vi "S7-TCP_Write.vi"(5 "DataType":T1=enum."Dword", 7 "DB #":u16=1, 8 "error in (no error)":errorcluster caption="错误输入（无错误）", 9 "WriteData":sgl[](array[numeric]), 10 "WriteAddress":sgl format="%#.1g", 11 "S7-TCP 输入":refnum<class "S7-TCP.lvclass">) -> (0 "error out":errorcluster caption="错误输出", 2 "Data Valid":bool, 3 "S7-TCP 输出":refnum<class "S7-TCP.lvclass">)   [LabVIEW 2018, in "S7-TCP.lvclass"]
uses:
  S7-TCP.lvclass
  Controls/WriteDataType.ctl
  Controls/RegisterType.ctl
  S7-TCP.lvclass/S7-TCP.ctl
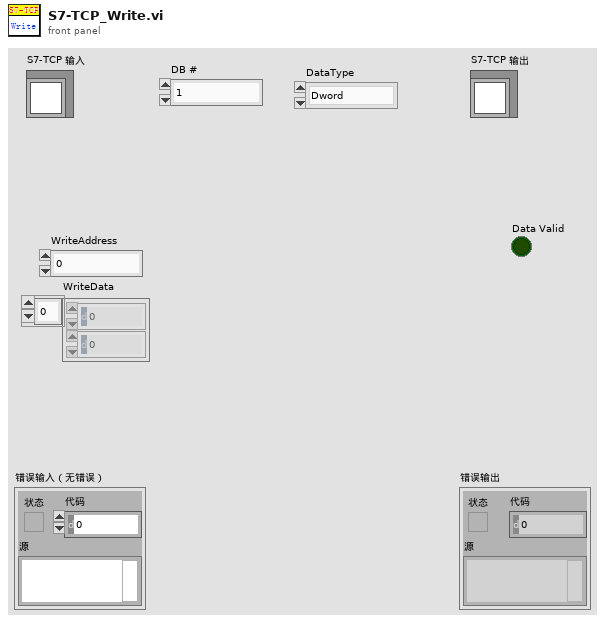
[diagram p1: front panel]
types:
  T1 = typedef "S7-TCP.lvclass/WriteDataType.ctl" = enum16{"Byte", "Word", "Dword", "Real", "Bit"}
  T2 = typedef "S7-TCP.lvclass/RegisterType.ctl" = u8
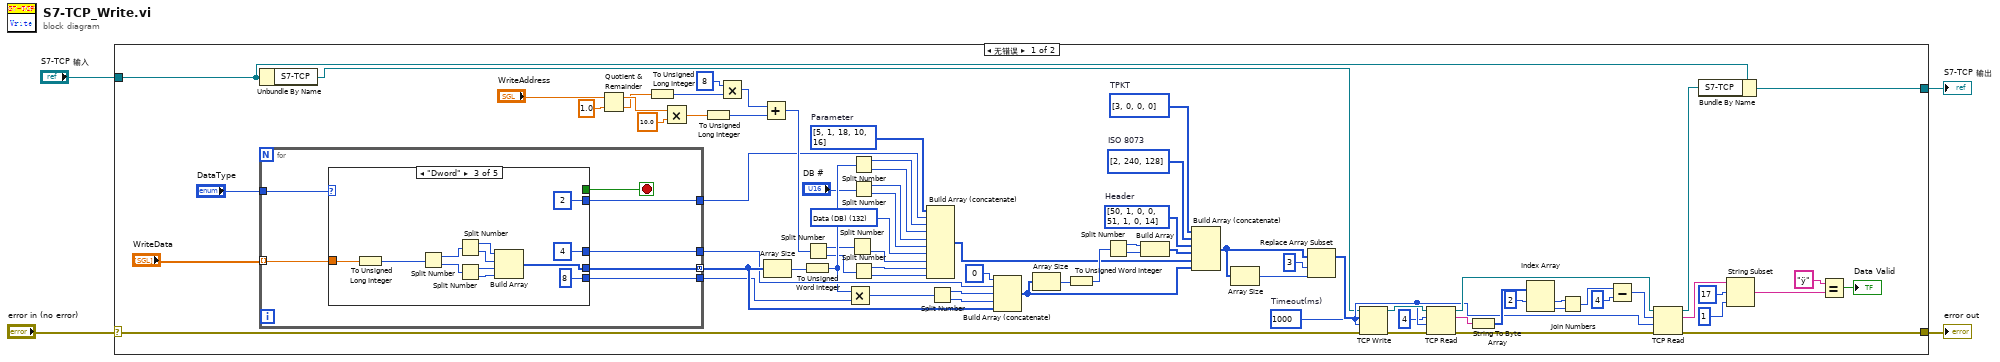
[diagram p0: block diagram]
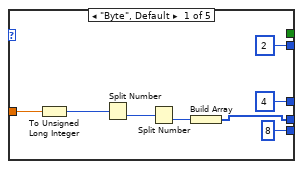
[diagram p2: hidden frame]
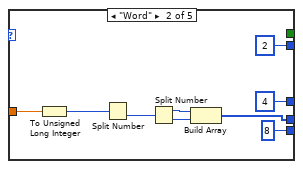
[diagram p3: hidden frame]
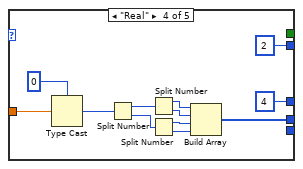
[diagram p4: hidden frame]
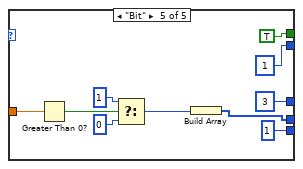
[diagram p5: hidden frame]
diagram:
  n1 = case shown="无错误" "error in (no error)" {
    selector: "error in (no error)" -> [w9 w139]
    tunnel: [w5 w139] -> w3
    tunnel: [w7 w138] -> w1
    tunnel: "S7-TCP 输入" -> [w79 w138]
    frame No Error {
      w12 = T2 132 items=["I/O (P)"=128, "Input (I)"=129, "Output (Q)"=130, "Bit Memory (M)"=131, "Data (DB)"=132, "Instance Data (DI)"=133, "Local Data (L)"=134, "Predecessor Local Data (VL)"=135] ("RegisterType")
      w24 = u32 1000  # Timeout(ms)
      w16 = u8[] [50, 1, 0, 0, 51, 1, 0, 14]  # Header
      w18 = u8[] [3, 0, 0, 0]  # TPKT
      w17 = u8[] [2, 240, 128]  # ISO 8073
      w13 = u8[] [5, 1, 18, 10, 16]  # Parameter
      n2 = Unbundle By Name(w79) -> ("S7-TCP"=w8:refnum<k5>)
      n3 = for {
        tunnel: "DataType" -> [w86]
        tunnel: "WriteData" -> [w85] mode=indexing
        tunnel: [w80] -> w78 mode=concatenating
        tunnel: [w84] -> w49
        tunnel: [w83] -> w63
        tunnel: [w82] -> w64
        stop <- w81 stop-if-true
        n4 = case shown="\"Dword\"" w86 {
          tunnel: w85 -> [w93 w100 w108 w118 w137]
          tunnel: [w94 w103 w109 w119 w132] -> w80
          tunnel: [u8 2 ("Numeric") u8 2 ("Numeric") u8 2 ("Numeric") u8 2 ("Numeric") u8 1 ("Numeric")] -> w84
          tunnel: [u8 4 ("Numeric") u8 4 ("Numeric") u8 4 ("Numeric") u8 4 ("Numeric") u8 3 ("Numeric")] -> w83
          tunnel: [u8 8 ("y") u8 8 ("y") u8 8 ("y") _ u16 1 ("y")] -> w82
          tunnel: [_ _ _ _ TRUE] -> w81
          frame "Byte", Default {
            n5 = To Unsigned Long Integer(number=w93) -> (unsigned 32bit integer=w91:u32)
            n6 = Split Number(x=w91) -> (lo(x)=w92:u16)  [unwired: 1 out]
            n7 = Split Number(x=w92) -> (lo(x)=w90:u8)  [unwired: 1 out]
            n8 = Build Array(w90) -> (w94:u8[])
          }
          frame "Word" {
            n9 = To Unsigned Long Integer(number=w100) -> (unsigned 32bit integer=w99:u32)
            n10 = Split Number(x=w99) -> (lo(x)=w98:u16)  [unwired: 1 out]
            n11 = Split Number(x=w98) -> (hi(x)=w102:u8, lo(x)=w101:u8)
            n12 = Build Array(w102, w101) -> (w103:u8[])
          }
          frame "Dword" {
            n13 = To Unsigned Long Integer(number=w108) -> (unsigned 32bit integer=w107:u32)
            n14 = Split Number(x=w107) -> (hi(x)=w115:u16, lo(x)=w114:u16)
            n15 = Split Number(x=w115) -> (hi(x)=w113:u8, lo(x)=w112:u8)
            n16 = Split Number(x=w114) -> (hi(x)=w111:u8, lo(x)=w110:u8)
            n17 = Build Array(w113, w112, w111, w110) -> (w109:u8[])
          }
          frame "Real" {
            n18 = Type Cast ("强制类型转换")(type=u32 0, x=w118) -> (*(type *) &x=w124:u32)
            n19 = Split Number(x=w124) -> (hi(x)=w126:u16, lo(x)=w125:u16)
            n20 = Split Number(x=w126) -> (hi(x)=w123:u8, lo(x)=w122:u8)
            n21 = Split Number(x=w125) -> (hi(x)=w121:u8, lo(x)=w120:u8)
            n22 = Build Array(w123, w122, w121, w120) -> (w119:u8[])
          }
          frame "Bit" {
            n23 = Greater Than 0?(x=w137) -> (x > 0?=w136:bool)
            n24 = Select(t=u8 1, s=w136, f=u8 0) -> (s? t:f=w133:u8)
            n25 = Build Array(w133) -> (w132:u8[])
          }
        }
      }
      n26 = Quotient & Remainder(x="WriteAddress", y=sgl 1.0) -> (x-y*floor(x/y)=w76:sgl, floor(x/y)=w75:sgl)
      n27 = To Unsigned Long Integer(number=w75) -> (unsigned 32bit integer=w53:u32)
      n28 = Multiply(x=w76, y=sgl 10.0) -> (x*y=w54:sgl)
      n29 = To Unsigned Long Integer(number=w54) -> (unsigned 32bit integer=w55:u32)
      n30 = Multiply(x=u32 8 ("y"), y=w53) -> (x*y=w51:u32)
      n31 = Add(x=w51, y=w55) -> (x+y=w52:u32)
      n32 = Array Size(array=w78) -> (size(s)=w42:i32)
      n33 = To Unsigned Word Integer(number=w42) -> (unsigned 16bit integer=w47:u16)
      n34 = Split Number(x=w52) -> (hi(x)=w34:u16, lo(x)=w35:u16)
      n35 = Multiply(x=w47, y=w64) -> (x*y=w44:u16)
      n36 = Split Number(x=w34) -> (lo(x)=w50:u8)  [unwired: 1 out]
      n37 = Split Number(x=w47) -> (hi(x)=w36:u8, lo(x)=w41:u8)
      n38 = Split Number(x="DB #") -> (hi(x)=w40:u8, lo(x)=w39:u8)
      n39 = Split Number(x=w35) -> (hi(x)=w37:u8, lo(x)=w38:u8)
      n40 = Build Array (concatenate)(w13, w49, w36, w41, w40, w39, w12, w50, w37, w38) -> (w56:T2[])
      n41 = Split Number(x=w44) -> (hi(x)=w46:u8, lo(x)=w45:u8)
      n42 = Build Array (concatenate)(u8 0 ("DLE"), w63, w46, w45, w78) -> (w57:u8[])
      n43 = Array Size(array=w57) -> (size(s)=w61:i32)
      n44 = To Unsigned Word Integer(number=w61) -> (unsigned 16bit integer=w62:u16)
      n45 = Split Number(x=w62) -> (hi(x)=w58:u8, lo(x)=w59:u8)
      n46 = Build Array(w58, w59) -> (w60:u8[])
      n47 = Build Array (concatenate)(w18, w17, w16, w60, w56, w57) -> (w48:T2[])
      n48 = Array Size(array=w48) -> (size(s)=w33:i32)
      n49 = Replace Array Subset(array=w48, new element=w33, index=3) -> (w43:T2[])
      n50 = TCP Write(connection ID=w8, data in=w43, error in (no error)=w9, 9:w24) -> (connection ID out=w31:refnum<k5>, error out=w32:errorcluster)  [unwired: 1 out]
      n51 = TCP Read(connection ID=w31, bytes to read=4, error in (no error)=w32, 9:w24) -> (connection ID out=w66:refnum<k5>, data out=w69:string, error out=w67:errorcluster)  [unwired: 1 in]
      n52 = String To Byte Array(string=w69) -> (unsigned byte array=w70:u8[])
      n53 = Index Array(array=w70, index #1=2 ("索引")) -> (element #1=w71:u8, element #2=w72:u8)  [unwired: 1 in]
      n54 = Join Numbers(hi=w71, lo=w72) -> ((hi.lo)=w73:u16)
      n55 = Subtract(x=w73, y=u16 4) -> (x-y=w74:u16)
      n56 = TCP Read(connection ID=w66, bytes to read=w74, error in (no error)=w67, 9:w24) -> (connection ID out=w6:refnum<k5>, data out=w68:string, error out=w5:errorcluster)  [unwired: 1 in]
      n57 = Bundle By Name(cluster=w79, "S7-TCP"=w6) -> (w7:refnum<class "S7-TCP.lvclass">)
      n58 = String Subset(string=w68, offset (0)=17 ("偏移量(0)"), length (rest)=1 ("长度（剩余）")) -> (substring=w65:string)
      n59 = Equal?(x="ÿ", y=w65) -> (x = y?=→"Data Valid":bool)
    }
    frame Error {
    }
  }
  "error out" <- w3
  "S7-TCP 输出" <- w1
